vi "Write wires.vi"(5 "wires":refnum<class "Wire.lvclass">[](array[class]), 9 "Diagram in":refnum<class "Diagram.lvclass">) -> (3 "Diagram out":refnum<class "Diagram.lvclass">)   [LabVIEW 2014, in "Raspberry Pi Compatible Compiler for LabVIEW.lvlib" / "Diagram.lvclass"]
uses:
  Diagram.lvclass
  Wire/Wire.lvclass
  Diagram.lvclass/Diagram.ctl
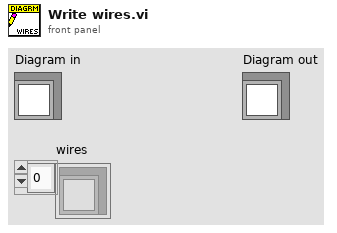
[diagram p1: front panel]
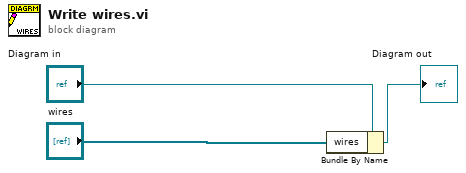
[diagram p0: block diagram]
diagram:
  n1 = Bundle By Name(cluster="Diagram in", "wires"="wires") -> (→"Diagram out":refnum<class "Diagram.lvclass">)
